vi "Color Sensor V3 Close.vi"(8 "error in (no error)":errorcluster, 11 "ColorSensorDevRef in":T1 {"I2CDevRef"."Device Address" format="%.0x"}) -> (0 "error out":errorcluster)   [LabVIEW 2019]
uses:
  <vilib>/Rock Robotics/WPI/ThirdParty/REV Robotics/Color SensorV3/Typedef/Color Sensor V3 DevRef.ctl
  <vilib>/Rock Robotics/WPI/I2C/WPI_I2CDevRef.ctl
  <vilib>/Rock Robotics/SystemInterfaces/i2clib/i2c_bus.ctl
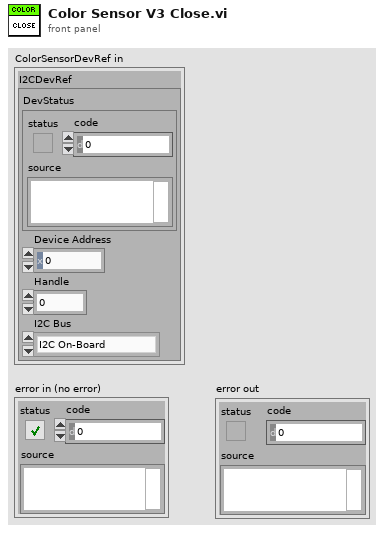
[diagram p1: front panel]
types:
  T1 = typedef "Color Sensor V3 DevRef.ctl" = cluster{"I2CDevRef":T2}
  T2 = typedef "WPI_I2CDevRef.ctl" = cluster{"DevStatus":errorcluster, "Device Address":u8, "Handle":i32, "I2C Bus":T3}
  T3 = typedef "i2c_bus.ctl" = enum16{"I2C On-Board", "I2C MXP", "Invalid"}
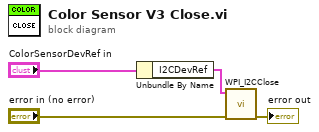
[diagram p0: block diagram]
diagram:
  n1 = Unbundle By Name("ColorSensorDevRef in") -> ("I2CDevRef"=w2:T2)
  n2 = call <vilib>:"WPI_I2CClose.vi"("error in (no error)"="error in (no error)", "I2CDevRef"=w2) -> ("error out"=→"error out":errorcluster)  [unwired: 9 in]
